vi "WILT Valve Test.vi"(0 "Water Valves Cluster":T8, 1 "Test Type":T7=enum."Full Valve Control", 2 "Operation Type":T11=enum."Operate As Stand-Alone EXE", 3 "Valve ON Time":dbl=100.0, 5 "Start Buttons Cluster":T9, 7 "Station Test State In":T5, 9 "Station Number":i32, 11 "Error In":errorcluster, 12 "Injection Times":T4, 13 "Day/Night Cycle":T10) -> (4 "Valve Actuation Complete":bool, 6 "Test Station Out":T5, 15 "Error Out":errorcluster)   [LabVIEW 2016] (continued)
                  tunnel: [T9 {"Start Button 21"=FALSE, "Start Button 22"=FALSE, "Start Button 23"=FALSE, "Start Button 24"=FALSE, "Start Button 25"=FALSE, "Start Button 26"=FALSE, "Start Button 27"=FALSE, "Start Button 28"=FALSE, "Start Button 29"=FALSE, "Start Button 30"=FALSE, "Start Button 31"=FALSE, "Start Button 32"=FALSE, "Start Button 33"=FALSE, "Start Button 34"=FALSE, "Start Button 35"=FALSE, "Start Button 36"=FALSE, "Start Button 37"=FALSE, "Start Button 38"=FALSE, "Start Button 39"=FALSE, "Start Button 40"=FALSE, "Start Button 41"=FALSE, "Start Button 42"=FALSE, "Start Button 43"=FALSE, "Start Button 44"=FALSE, "Start Button 12"=FALSE, "Start Button 11"=FALSE, "Start Button 10"=FALSE, "Start Button 9"=FALSE, "Start Button 8"=FALSE, "Start Button 7"=FALSE, "Start Button 6"=FALSE, "Start Button 5"=FALSE, "Start Button 4"=FALSE, "Start Button 3"=FALSE, "Start Button 2"=FALSE, "Start Button 1"=FALSE, "Start Button 20"=FALSE, "Start Button 19"=FALSE, "Start Button 18"=FALSE, "Start Button 17"=FALSE, "Start Button 16"=FALSE, "Start Button 15"=FALSE, "Start Button 14"=FALSE, "Start Button 13"=FALSE, "Start Button 45"=FALSE, "Start Button 46"=FALSE, "Start Button 47"=FALSE, "Start Button 48"=FALSE, "Start Button 49"=FALSE, "Start Button 50"=FALSE, "Start Button 51"=FALSE, "Start Button 52"=FALSE, "Start Button 53"=FALSE, "Start Button 54"=FALSE, "Start Button 55"=FALSE, "Start Button 56"=FALSE} ("Start Buttons Cluster") T9 {"Start Button 21"=FALSE, "Start Button 22"=FALSE, "Start Button 23"=FALSE, "Start Button 24"=FALSE, "Start Button 25"=FALSE, "Start Button 26"=FALSE, "Start Button 27"=FALSE, "Start Button 28"=FALSE, "Start Button 29"=FALSE, "Start Button 30"=FALSE, "Start Button 31"=FALSE, "Start Button 32"=FALSE, "Start Button 33"=FALSE, "Start Button 34"=FALSE, "Start Button 35"=FALSE, "Start Button 36"=FALSE, "Start Button 37"=FALSE, "Start Button 38"=FALSE, "Start Button 39"=FALSE, "Start Button 40"=FALSE, "Start Button 41"=FALSE, "Start Button 42"=FALSE, "Start Button 43"=FALSE, "Start Button 44"=FALSE, "Start Button 12"=FALSE, "Start Button 11"=FALSE, "Start Button 10"=FALSE, "Start Button 9"=FALSE, "Start Button 8"=FALSE, "Start Button 7"=FALSE, "Start Button 6"=FALSE, "Start Button 5"=FALSE, "Start Button 4"=FALSE, "Start Button 3"=FALSE, "Start Button 2"=FALSE, "Start Button 1"=FALSE, "Start Button 20"=FALSE, "Start Button 19"=FALSE, "Start Button 18"=FALSE, "Start Button 17"=FALSE, "Start Button 16"=FALSE, "Start Button 15"=FALSE, "Start Button 14"=FALSE, "Start Button 13"=FALSE, "Start Button 45"=FALSE, "Start Button 46"=FALSE, "Start Button 47"=FALSE, "Start Button 48"=FALSE, "Start Button 49"=FALSE, "Start Button 50"=FALSE, "Start Button 51"=FALSE, "Start Button 52"=FALSE, "Start Button 53"=FALSE, "Start Button 54"=FALSE, "Start Button 55"=FALSE, "Start Button 56"=FALSE} ("Start Buttons Cluster") w1471 w1474 w1478] -> w1458
                  frame "Water Injection 1 (On)", Default {
                    n436 = Bundle By Name(cluster=T8 {"Valve 1"=FALSE, "Valve 2"=FALSE, "Valve 3"=FALSE, "Valve 4"=FALSE, "Valve 5"=FALSE, "Valve 6"=FALSE, "Valve 7"=FALSE, "Valve 8"=FALSE, "Valve 9"=FALSE, "Valve 10"=FALSE, "Valve 11"=FALSE, "Valve 12"=FALSE, "Valve 13"=FALSE, "Valve 14"=FALSE, "Valve 15"=FALSE, "Valve 16"=FALSE, "Valve 17"=FALSE, "Valve 18"=FALSE, "Valve 19"=FALSE, "Valve 20"=FALSE, "Valve 21"=FALSE, "Valve 22"=FALSE, "Valve 23"=FALSE, "Valve 24"=FALSE, "Valve 25"=FALSE, "Valve 26"=FALSE, "Valve 27"=FALSE, "Valve 28"=FALSE, "Valve 29"=FALSE, "Valve 30"=FALSE, "Valve 31"=FALSE, "Valve 32"=FALSE, "Valve 33"=FALSE, "Valve 34"=FALSE, "Valve 35"=FALSE, "Valve 36"=FALSE, "Valve 37"=FALSE, "Valve 38"=FALSE, "Valve 39"=FALSE, "Valve 40"=FALSE, "Valve 41"=FALSE, "Valve 42"=FALSE, "Valve 43"=FALSE, "Valve 44"=FALSE, "Valve 45"=FALSE, "Valve 46"=FALSE, "Valve 47"=FALSE, "Valve 48"=FALSE, "Valve 49"=FALSE, "Valve 50"=FALSE, "Valve 51"=FALSE, "Valve 52"=FALSE, "Valve 53"=FALSE, "Valve 54"=FALSE, "Valve 55"=FALSE, "Valve 56"=FALSE} ("Water Valves Cluster"), "Valve 54"=TRUE ("Valve 1")) -> (w1463:T8)
                  }
                  frame "Drying Clothes 2" {
                    n437 = Bundle By Name(cluster=T8 {"Valve 1"=FALSE, "Valve 2"=FALSE, "Valve 3"=FALSE, "Valve 4"=FALSE, "Valve 5"=FALSE, "Valve 6"=FALSE, "Valve 7"=FALSE, "Valve 8"=FALSE, "Valve 9"=FALSE, "Valve 10"=FALSE, "Valve 11"=FALSE, "Valve 12"=FALSE, "Valve 13"=FALSE, "Valve 14"=FALSE, "Valve 15"=FALSE, "Valve 16"=FALSE, "Valve 17"=FALSE, "Valve 18"=FALSE, "Valve 19"=FALSE, "Valve 20"=FALSE, "Valve 21"=FALSE, "Valve 22"=FALSE, "Valve 23"=FALSE, "Valve 24"=FALSE, "Valve 25"=FALSE, "Valve 26"=FALSE, "Valve 27"=FALSE, "Valve 28"=FALSE, "Valve 29"=FALSE, "Valve 30"=FALSE, "Valve 31"=FALSE, "Valve 32"=FALSE, "Valve 33"=FALSE, "Valve 34"=FALSE, "Valve 35"=FALSE, "Valve 36"=FALSE, "Valve 37"=FALSE, "Valve 38"=FALSE, "Valve 39"=FALSE, "Valve 40"=FALSE, "Valve 41"=FALSE, "Valve 42"=FALSE, "Valve 43"=FALSE, "Valve 44"=FALSE, "Valve 45"=FALSE, "Valve 46"=FALSE, "Valve 47"=FALSE, "Valve 48"=FALSE, "Valve 49"=FALSE, "Valve 50"=FALSE, "Valve 51"=FALSE, "Valve 52"=FALSE, "Valve 53"=FALSE, "Valve 54"=FALSE, "Valve 55"=FALSE, "Valve 56"=FALSE} ("Water Valves Cluster"), "Valve 54"=TRUE ("Valve 1")) -> (w1467:T8)
                  }
                  frame "Sending Start Stop CMD" {
                    n438 = Bundle By Name(cluster=T9 {"Start Button 21"=FALSE, "Start Button 22"=FALSE, "Start Button 23"=FALSE, "Start Button 24"=FALSE, "Start Button 25"=FALSE, "Start Button 26"=FALSE, "Start Button 27"=FALSE, "Start Button 28"=FALSE, "Start Button 29"=FALSE, "Start Button 30"=FALSE, "Start Button 31"=FALSE, "Start Button 32"=FALSE, "Start Button 33"=FALSE, "Start Button 34"=FALSE, "Start Button 35"=FALSE, "Start Button 36"=FALSE, "Start Button 37"=FALSE, "Start Button 38"=FALSE, "Start Button 39"=FALSE, "Start Button 40"=FALSE, "Start Button 41"=FALSE, "Start Button 42"=FALSE, "Start Button 43"=FALSE, "Start Button 44"=FALSE, "Start Button 12"=FALSE, "Start Button 11"=FALSE, "Start Button 10"=FALSE, "Start Button 9"=FALSE, "Start Button 8"=FALSE, "Start Button 7"=FALSE, "Start Button 6"=FALSE, "Start Button 5"=FALSE, "Start Button 4"=FALSE, "Start Button 3"=FALSE, "Start Button 2"=FALSE, "Start Button 1"=FALSE, "Start Button 20"=FALSE, "Start Button 19"=FALSE, "Start Button 18"=FALSE, "Start Button 17"=FALSE, "Start Button 16"=FALSE, "Start Button 15"=FALSE, "Start Button 14"=FALSE, "Start Button 13"=FALSE, "Start Button 45"=FALSE, "Start Button 46"=FALSE, "Start Button 47"=FALSE, "Start Button 48"=FALSE, "Start Button 49"=FALSE, "Start Button 50"=FALSE, "Start Button 51"=FALSE, "Start Button 52"=FALSE, "Start Button 53"=FALSE, "Start Button 54"=FALSE, "Start Button 55"=FALSE, "Start Button 56"=FALSE} ("Start Buttons Cluster"), "Start Button 54"=TRUE ("Start Button 21")) -> (w1471:T9)
                  }
                  frame "Sending Start Stop CMD 2" {
                    n439 = Bundle By Name(cluster=T9 {"Start Button 21"=FALSE, "Start Button 22"=FALSE, "Start Button 23"=FALSE, "Start Button 24"=FALSE, "Start Button 25"=FALSE, "Start Button 26"=FALSE, "Start Button 27"=FALSE, "Start Button 28"=FALSE, "Start Button 29"=FALSE, "Start Button 30"=FALSE, "Start Button 31"=FALSE, "Start Button 32"=FALSE, "Start Button 33"=FALSE, "Start Button 34"=FALSE, "Start Button 35"=FALSE, "Start Button 36"=FALSE, "Start Button 37"=FALSE, "Start Button 38"=FALSE, "Start Button 39"=FALSE, "Start Button 40"=FALSE, "Start Button 41"=FALSE, "Start Button 42"=FALSE, "Start Button 43"=FALSE, "Start Button 44"=FALSE, "Start Button 12"=FALSE, "Start Button 11"=FALSE, "Start Button 10"=FALSE, "Start Button 9"=FALSE, "Start Button 8"=FALSE, "Start Button 7"=FALSE, "Start Button 6"=FALSE, "Start Button 5"=FALSE, "Start Button 4"=FALSE, "Start Button 3"=FALSE, "Start Button 2"=FALSE, "Start Button 1"=FALSE, "Start Button 20"=FALSE, "Start Button 19"=FALSE, "Start Button 18"=FALSE, "Start Button 17"=FALSE, "Start Button 16"=FALSE, "Start Button 15"=FALSE, "Start Button 14"=FALSE, "Start Button 13"=FALSE, "Start Button 45"=FALSE, "Start Button 46"=FALSE, "Start Button 47"=FALSE, "Start Button 48"=FALSE, "Start Button 49"=FALSE, "Start Button 50"=FALSE, "Start Button 51"=FALSE, "Start Button 52"=FALSE, "Start Button 53"=FALSE, "Start Button 54"=FALSE, "Start Button 55"=FALSE, "Start Button 56"=FALSE} ("Start Buttons Cluster"), "Start Button 54"=TRUE ("Start Button 21")) -> (w1474:T9)
                  }
                  frame "Sending Start Stop CMD 3" {
                    n440 = Bundle By Name(cluster=T9 {"Start Button 21"=FALSE, "Start Button 22"=FALSE, "Start Button 23"=FALSE, "Start Button 24"=FALSE, "Start Button 25"=FALSE, "Start Button 26"=FALSE, "Start Button 27"=FALSE, "Start Button 28"=FALSE, "Start Button 29"=FALSE, "Start Button 30"=FALSE, "Start Button 31"=FALSE, "Start Button 32"=FALSE, "Start Button 33"=FALSE, "Start Button 34"=FALSE, "Start Button 35"=FALSE, "Start Button 36"=FALSE, "Start Button 37"=FALSE, "Start Button 38"=FALSE, "Start Button 39"=FALSE, "Start Button 40"=FALSE, "Start Button 41"=FALSE, "Start Button 42"=FALSE, "Start Button 43"=FALSE, "Start Button 44"=FALSE, "Start Button 12"=FALSE, "Start Button 11"=FALSE, "Start Button 10"=FALSE, "Start Button 9"=FALSE, "Start Button 8"=FALSE, "Start Button 7"=FALSE, "Start Button 6"=FALSE, "Start Button 5"=FALSE, "Start Button 4"=FALSE, "Start Button 3"=FALSE, "Start Button 2"=FALSE, "Start Button 1"=FALSE, "Start Button 20"=FALSE, "Start Button 19"=FALSE, "Start Button 18"=FALSE, "Start Button 17"=FALSE, "Start Button 16"=FALSE, "Start Button 15"=FALSE, "Start Button 14"=FALSE, "Start Button 13"=FALSE, "Start Button 45"=FALSE, "Start Button 46"=FALSE, "Start Button 47"=FALSE, "Start Button 48"=FALSE, "Start Button 49"=FALSE, "Start Button 50"=FALSE, "Start Button 51"=FALSE, "Start Button 52"=FALSE, "Start Button 53"=FALSE, "Start Button 54"=FALSE, "Start Button 55"=FALSE, "Start Button 56"=FALSE} ("Start Buttons Cluster"), "Start Button 54"=TRUE ("Start Button 21")) -> (w1478:T9)
                  }
                }
              }
              frame 55 {
                n441 = Unbundle By Name(w1485) -> ("Station Test State 55"=w1484:T6)
                n442 = case shown="\"Sending Start Stop CMD 3\"" w1484 {
                  tunnel: [w1487 w1491 T8 {"Valve 1"=FALSE, "Valve 2"=FALSE, "Valve 3"=FALSE, "Valve 4"=FALSE, "Valve 5"=FALSE, "Valve 6"=FALSE, "Valve 7"=FALSE, "Valve 8"=FALSE, "Valve 9"=FALSE, "Valve 10"=FALSE, "Valve 11"=FALSE, "Valve 12"=FALSE, "Valve 13"=FALSE, "Valve 14"=FALSE, "Valve 15"=FALSE, "Valve 16"=FALSE, "Valve 17"=FALSE, "Valve 18"=FALSE, "Valve 19"=FALSE, "Valve 20"=FALSE, "Valve 21"=FALSE, "Valve 22"=FALSE, "Valve 23"=FALSE, "Valve 24"=FALSE, "Valve 25"=FALSE, "Valve 26"=FALSE, "Valve 27"=FALSE, "Valve 28"=FALSE, "Valve 29"=FALSE, "Valve 30"=FALSE, "Valve 31"=FALSE, "Valve 32"=FALSE, "Valve 33"=FALSE, "Valve 34"=FALSE, "Valve 35"=FALSE, "Valve 36"=FALSE, "Valve 37"=FALSE, "Valve 38"=FALSE, "Valve 39"=FALSE, "Valve 40"=FALSE, "Valve 41"=FALSE, "Valve 42"=FALSE, "Valve 43"=FALSE, "Valve 44"=FALSE, "Valve 45"=FALSE, "Valve 46"=FALSE, "Valve 47"=FALSE, "Valve 48"=FALSE, "Valve 49"=FALSE, "Valve 50"=FALSE, "Valve 51"=FALSE, "Valve 52"=FALSE, "Valve 53"=FALSE, "Valve 54"=FALSE, "Valve 55"=FALSE, "Valve 56"=FALSE} ("Water Valves Cluster") T8 {"Valve 1"=FALSE, "Valve 2"=FALSE, "Valve 3"=FALSE, "Valve 4"=FALSE, "Valve 5"=FALSE, "Valve 6"=FALSE, "Valve 7"=FALSE, "Valve 8"=FALSE, "Valve 9"=FALSE, "Valve 10"=FALSE, "Valve 11"=FALSE, "Valve 12"=FALSE, "Valve 13"=FALSE, "Valve 14"=FALSE, "Valve 15"=FALSE, "Valve 16"=FALSE, "Valve 17"=FALSE, "Valve 18"=FALSE, "Valve 19"=FALSE, "Valve 20"=FALSE, "Valve 21"=FALSE, "Valve 22"=FALSE, "Valve 23"=FALSE, "Valve 24"=FALSE, "Valve 25"=FALSE, "Valve 26"=FALSE, "Valve 27"=FALSE, "Valve 28"=FALSE, "Valve 29"=FALSE, "Valve 30"=FALSE, "Valve 31"=FALSE, "Valve 32"=FALSE, "Valve 33"=FALSE, "Valve 34"=FALSE, "Valve 35"=FALSE, "Valve 36"=FALSE, "Valve 37"=FALSE, "Valve 38"=FALSE, "Valve 39"=FALSE, "Valve 40"=FALSE, "Valve 41"=FALSE, "Valve 42"=FALSE, "Valve 43"=FALSE, "Valve 44"=FALSE, "Valve 45"=FALSE, "Valve 46"=FALSE, "Valve 47"=FALSE, "Valve 48"=FALSE, "Valve 49"=FALSE, "Valve 50"=FALSE, "Valve 51"=FALSE, "Valve 52"=FALSE, "Valve 53"=FALSE, "Valve 54"=FALSE, "Valve 55"=FALSE, "Valve 56"=FALSE} ("Water Valves Cluster") T8 {"Valve 1"=FALSE, "Valve 2"=FALSE, "Valve 3"=FALSE, "Valve 4"=FALSE, "Valve 5"=FALSE, "Valve 6"=FALSE, "Valve 7"=FALSE, "Valve 8"=FALSE, "Valve 9"=FALSE, "Valve 10"=FALSE, "Valve 11"=FALSE, "Valve 12"=FALSE, "Valve 13"=FALSE, "Valve 14"=FALSE, "Valve 15"=FALSE, "Valve 16"=FALSE, "Valve 17"=FALSE, "Valve 18"=FALSE, "Valve 19"=FALSE, "Valve 20"=FALSE, "Valve 21"=FALSE, "Valve 22"=FALSE, "Valve 23"=FALSE, "Valve 24"=FALSE, "Valve 25"=FALSE, "Valve 26"=FALSE, "Valve 27"=FALSE, "Valve 28"=FALSE, "Valve 29"=FALSE, "Valve 30"=FALSE, "Valve 31"=FALSE, "Valve 32"=FALSE, "Valve 33"=FALSE, "Valve 34"=FALSE, "Valve 35"=FALSE, "Valve 36"=FALSE, "Valve 37"=FALSE, "Valve 38"=FALSE, "Valve 39"=FALSE, "Valve 40"=FALSE, "Valve 41"=FALSE, "Valve 42"=FALSE, "Valve 43"=FALSE, "Valve 44"=FALSE, "Valve 45"=FALSE, "Valve 46"=FALSE, "Valve 47"=FALSE, "Valve 48"=FALSE, "Valve 49"=FALSE, "Valve 50"=FALSE, "Valve 51"=FALSE, "Valve 52"=FALSE, "Valve 53"=FALSE, "Valve 54"=FALSE, "Valve 55"=FALSE, "Valve 56"=FALSE} ("Water Valves Cluster")] -> w1483
                  tunnel: [T9 {"Start Button 21"=FALSE, "Start Button 22"=FALSE, "Start Button 23"=FALSE, "Start Button 24"=FALSE, "Start Button 25"=FALSE, "Start Button 26"=FALSE, "Start Button 27"=FALSE, "Start Button 28"=FALSE, "Start Button 29"=FALSE, "Start Button 30"=FALSE, "Start Button 31"=FALSE, "Start Button 32"=FALSE, "Start Button 33"=FALSE, "Start Button 34"=FALSE, "Start Button 35"=FALSE, "Start Button 36"=FALSE, "Start Button 37"=FALSE, "Start Button 38"=FALSE, "Start Button 39"=FALSE, "Start Button 40"=FALSE, "Start Button 41"=FALSE, "Start Button 42"=FALSE, "Start Button 43"=FALSE, "Start Button 44"=FALSE, "Start Button 12"=FALSE, "Start Button 11"=FALSE, "Start Button 10"=FALSE, "Start Button 9"=FALSE, "Start Button 8"=FALSE, "Start Button 7"=FALSE, "Start Button 6"=FALSE, "Start Button 5"=FALSE, "Start Button 4"=FALSE, "Start Button 3"=FALSE, "Start Button 2"=FALSE, "Start Button 1"=FALSE, "Start Button 20"=FALSE, "Start Button 19"=FALSE, "Start Button 18"=FALSE, "Start Button 17"=FALSE, "Start Button 16"=FALSE, "Start Button 15"=FALSE, "Start Button 14"=FALSE, "Start Button 13"=FALSE, "Start Button 45"=FALSE, "Start Button 46"=FALSE, "Start Button 47"=FALSE, "Start Button 48"=FALSE, "Start Button 49"=FALSE, "Start Button 50"=FALSE, "Start Button 51"=FALSE, "Start Button 52"=FALSE, "Start Button 53"=FALSE, "Start Button 54"=FALSE, "Start Button 55"=FALSE, "Start Button 56"=FALSE} ("Start Buttons Cluster") T9 {"Start Button 21"=FALSE, "Start Button 22"=FALSE, "Start Button 23"=FALSE, "Start Button 24"=FALSE, "Start Button 25"=FALSE, "Start Button 26"=FALSE, "Start Button 27"=FALSE, "Start Button 28"=FALSE, "Start Button 29"=FALSE, "Start Button 30"=FALSE, "Start Button 31"=FALSE, "Start Button 32"=FALSE, "Start Button 33"=FALSE, "Start Button 34"=FALSE, "Start Button 35"=FALSE, "Start Button 36"=FALSE, "Start Button 37"=FALSE, "Start Button 38"=FALSE, "Start Button 39"=FALSE, "Start Button 40"=FALSE, "Start Button 41"=FALSE, "Start Button 42"=FALSE, "Start Button 43"=FALSE, "Start Button 44"=FALSE, "Start Button 12"=FALSE, "Start Button 11"=FALSE, "Start Button 10"=FALSE, "Start Button 9"=FALSE, "Start Button 8"=FALSE, "Start Button 7"=FALSE, "Start Button 6"=FALSE, "Start Button 5"=FALSE, "Start Button 4"=FALSE, "Start Button 3"=FALSE, "Start Button 2"=FALSE, "Start Button 1"=FALSE, "Start Button 20"=FALSE, "Start Button 19"=FALSE, "Start Button 18"=FALSE, "Start Button 17"=FALSE, "Start Button 16"=FALSE, "Start Button 15"=FALSE, "Start Button 14"=FALSE, "Start Button 13"=FALSE, "Start Button 45"=FALSE, "Start Button 46"=FALSE, "Start Button 47"=FALSE, "Start Button 48"=FALSE, "Start Button 49"=FALSE, "Start Button 50"=FALSE, "Start Button 51"=FALSE, "Start Button 52"=FALSE, "Start Button 53"=FALSE, "Start Button 54"=FALSE, "Start Button 55"=FALSE, "Start Button 56"=FALSE} ("Start Buttons Cluster") w1495 w1498 w1502] -> w1482
                  frame "Water Injection 1 (On)", Default {
                    n443 = Bundle By Name(cluster=T8 {"Valve 1"=FALSE, "Valve 2"=FALSE, "Valve 3"=FALSE, "Valve 4"=FALSE, "Valve 5"=FALSE, "Valve 6"=FALSE, "Valve 7"=FALSE, "Valve 8"=FALSE, "Valve 9"=FALSE, "Valve 10"=FALSE, "Valve 11"=FALSE, "Valve 12"=FALSE, "Valve 13"=FALSE, "Valve 14"=FALSE, "Valve 15"=FALSE, "Valve 16"=FALSE, "Valve 17"=FALSE, "Valve 18"=FALSE, "Valve 19"=FALSE, "Valve 20"=FALSE, "Valve 21"=FALSE, "Valve 22"=FALSE, "Valve 23"=FALSE, "Valve 24"=FALSE, "Valve 25"=FALSE, "Valve 26"=FALSE, "Valve 27"=FALSE, "Valve 28"=FALSE, "Valve 29"=FALSE, "Valve 30"=FALSE, "Valve 31"=FALSE, "Valve 32"=FALSE, "Valve 33"=FALSE, "Valve 34"=FALSE, "Valve 35"=FALSE, "Valve 36"=FALSE, "Valve 37"=FALSE, "Valve 38"=FALSE, "Valve 39"=FALSE, "Valve 40"=FALSE, "Valve 41"=FALSE, "Valve 42"=FALSE, "Valve 43"=FALSE, "Valve 44"=FALSE, "Valve 45"=FALSE, "Valve 46"=FALSE, "Valve 47"=FALSE, "Valve 48"=FALSE, "Valve 49"=FALSE, "Valve 50"=FALSE, "Valve 51"=FALSE, "Valve 52"=FALSE, "Valve 53"=FALSE, "Valve 54"=FALSE, "Valve 55"=FALSE, "Valve 56"=FALSE} ("Water Valves Cluster"), "Valve 55"=TRUE ("Valve 1")) -> (w1487:T8)
                  }
                  frame "Drying Clothes 2" {
                    n444 = Bundle By Name(cluster=T8 {"Valve 1"=FALSE, "Valve 2"=FALSE, "Valve 3"=FALSE, "Valve 4"=FALSE, "Valve 5"=FALSE, "Valve 6"=FALSE, "Valve 7"=FALSE, "Valve 8"=FALSE, "Valve 9"=FALSE, "Valve 10"=FALSE, "Valve 11"=FALSE, "Valve 12"=FALSE, "Valve 13"=FALSE, "Valve 14"=FALSE, "Valve 15"=FALSE, "Valve 16"=FALSE, "Valve 17"=FALSE, "Valve 18"=FALSE, "Valve 19"=FALSE, "Valve 20"=FALSE, "Valve 21"=FALSE, "Valve 22"=FALSE, "Valve 23"=FALSE, "Valve 24"=FALSE, "Valve 25"=FALSE, "Valve 26"=FALSE, "Valve 27"=FALSE, "Valve 28"=FALSE, "Valve 29"=FALSE, "Valve 30"=FALSE, "Valve 31"=FALSE, "Valve 32"=FALSE, "Valve 33"=FALSE, "Valve 34"=FALSE, "Valve 35"=FALSE, "Valve 36"=FALSE, "Valve 37"=FALSE, "Valve 38"=FALSE, "Valve 39"=FALSE, "Valve 40"=FALSE, "Valve 41"=FALSE, "Valve 42"=FALSE, "Valve 43"=FALSE, "Valve 44"=FALSE, "Valve 45"=FALSE, "Valve 46"=FALSE, "Valve 47"=FALSE, "Valve 48"=FALSE, "Valve 49"=FALSE, "Valve 50"=FALSE, "Valve 51"=FALSE, "Valve 52"=FALSE, "Valve 53"=FALSE, "Valve 54"=FALSE, "Valve 55"=FALSE, "Valve 56"=FALSE} ("Water Valves Cluster"), "Valve 55"=TRUE ("Valve 1")) -> (w1491:T8)
                  }
                  frame "Sending Start Stop CMD" {
                    n445 = Bundle By Name(cluster=T9 {"Start Button 21"=FALSE, "Start Button 22"=FALSE, "Start Button 23"=FALSE, "Start Button 24"=FALSE, "Start Button 25"=FALSE, "Start Button 26"=FALSE, "Start Button 27"=FALSE, "Start Button 28"=FALSE, "Start Button 29"=FALSE, "Start Button 30"=FALSE, "Start Button 31"=FALSE, "Start Button 32"=FALSE, "Start Button 33"=FALSE, "Start Button 34"=FALSE, "Start Button 35"=FALSE, "Start Button 36"=FALSE, "Start Button 37"=FALSE, "Start Button 38"=FALSE, "Start Button 39"=FALSE, "Start Button 40"=FALSE, "Start Button 41"=FALSE, "Start Button 42"=FALSE, "Start Button 43"=FALSE, "Start Button 44"=FALSE, "Start Button 12"=FALSE, "Start Button 11"=FALSE, "Start Button 10"=FALSE, "Start Button 9"=FALSE, "Start Button 8"=FALSE, "Start Button 7"=FALSE, "Start Button 6"=FALSE, "Start Button 5"=FALSE, "Start Button 4"=FALSE, "Start Button 3"=FALSE, "Start Button 2"=FALSE, "Start Button 1"=FALSE, "Start Button 20"=FALSE, "Start Button 19"=FALSE, "Start Button 18"=FALSE, "Start Button 17"=FALSE, "Start Button 16"=FALSE, "Start Button 15"=FALSE, "Start Button 14"=FALSE, "Start Button 13"=FALSE, "Start Button 45"=FALSE, "Start Button 46"=FALSE, "Start Button 47"=FALSE, "Start Button 48"=FALSE, "Start Button 49"=FALSE, "Start Button 50"=FALSE, "Start Button 51"=FALSE, "Start Button 52"=FALSE, "Start Button 53"=FALSE, "Start Button 54"=FALSE, "Start Button 55"=FALSE, "Start Button 56"=FALSE} ("Start Buttons Cluster"), "Start Button 55"=TRUE ("Start Button 21")) -> (w1495:T9)
                  }
                  frame "Sending Start Stop CMD 2" {
                    n446 = Bundle By Name(cluster=T9 {"Start Button 21"=FALSE, "Start Button 22"=FALSE, "Start Button 23"=FALSE, "Start Button 24"=FALSE, "Start Button 25"=FALSE, "Start Button 26"=FALSE, "Start Button 27"=FALSE, "Start Button 28"=FALSE, "Start Button 29"=FALSE, "Start Button 30"=FALSE, "Start Button 31"=FALSE, "Start Button 32"=FALSE, "Start Button 33"=FALSE, "Start Button 34"=FALSE, "Start Button 35"=FALSE, "Start Button 36"=FALSE, "Start Button 37"=FALSE, "Start Button 38"=FALSE, "Start Button 39"=FALSE, "Start Button 40"=FALSE, "Start Button 41"=FALSE, "Start Button 42"=FALSE, "Start Button 43"=FALSE, "Start Button 44"=FALSE, "Start Button 12"=FALSE, "Start Button 11"=FALSE, "Start Button 10"=FALSE, "Start Button 9"=FALSE, "Start Button 8"=FALSE, "Start Button 7"=FALSE, "Start Button 6"=FALSE, "Start Button 5"=FALSE, "Start Button 4"=FALSE, "Start Button 3"=FALSE, "Start Button 2"=FALSE, "Start Button 1"=FALSE, "Start Button 20"=FALSE, "Start Button 19"=FALSE, "Start Button 18"=FALSE, "Start Button 17"=FALSE, "Start Button 16"=FALSE, "Start Button 15"=FALSE, "Start Button 14"=FALSE, "Start Button 13"=FALSE, "Start Button 45"=FALSE, "Start Button 46"=FALSE, "Start Button 47"=FALSE, "Start Button 48"=FALSE, "Start Button 49"=FALSE, "Start Button 50"=FALSE, "Start Button 51"=FALSE, "Start Button 52"=FALSE, "Start Button 53"=FALSE, "Start Button 54"=FALSE, "Start Button 55"=FALSE, "Start Button 56"=FALSE} ("Start Buttons Cluster"), "Start Button 55"=TRUE ("Start Button 21")) -> (w1498:T9)
                  }
                  frame "Sending Start Stop CMD 3" {
                    n447 = Bundle By Name(cluster=T9 {"Start Button 21"=FALSE, "Start Button 22"=FALSE, "Start Button 23"=FALSE, "Start Button 24"=FALSE, "Start Button 25"=FALSE, "Start Button 26"=FALSE, "Start Button 27"=FALSE, "Start Button 28"=FALSE, "Start Button 29"=FALSE, "Start Button 30"=FALSE, "Start Button 31"=FALSE, "Start Button 32"=FALSE, "Start Button 33"=FALSE, "Start Button 34"=FALSE, "Start Button 35"=FALSE, "Start Button 36"=FALSE, "Start Button 37"=FALSE, "Start Button 38"=FALSE, "Start Button 39"=FALSE, "Start Button 40"=FALSE, "Start Button 41"=FALSE, "Start Button 42"=FALSE, "Start Button 43"=FALSE, "Start Button 44"=FALSE, "Start Button 12"=FALSE, "Start Button 11"=FALSE, "Start Button 10"=FALSE, "Start Button 9"=FALSE, "Start Button 8"=FALSE, "Start Button 7"=FALSE, "Start Button 6"=FALSE, "Start Button 5"=FALSE, "Start Button 4"=FALSE, "Start Button 3"=FALSE, "Start Button 2"=FALSE, "Start Button 1"=FALSE, "Start Button 20"=FALSE, "Start Button 19"=FALSE, "Start Button 18"=FALSE, "Start Button 17"=FALSE, "Start Button 16"=FALSE, "Start Button 15"=FALSE, "Start Button 14"=FALSE, "Start Button 13"=FALSE, "Start Button 45"=FALSE, "Start Button 46"=FALSE, "Start Button 47"=FALSE, "Start Button 48"=FALSE, "Start Button 49"=FALSE, "Start Button 50"=FALSE, "Start Button 51"=FALSE, "Start Button 52"=FALSE, "Start Button 53"=FALSE, "Start Button 54"=FALSE, "Start Button 55"=FALSE, "Start Button 56"=FALSE} ("Start Buttons Cluster"), "Start Button 55"=TRUE ("Start Button 21")) -> (w1502:T9)
                  }
                }
              }
              frame 56 {
                n448 = Unbundle By Name(w1509) -> ("Station Test State 56"=w1508:T6)
                n449 = case shown="\"Water Injection 1 (On)\", Default" w1508 {
                  tunnel: [w1511 w1515 T8 {"Valve 1"=FALSE, "Valve 2"=FALSE, "Valve 3"=FALSE, "Valve 4"=FALSE, "Valve 5"=FALSE, "Valve 6"=FALSE, "Valve 7"=FALSE, "Valve 8"=FALSE, "Valve 9"=FALSE, "Valve 10"=FALSE, "Valve 11"=FALSE, "Valve 12"=FALSE, "Valve 13"=FALSE, "Valve 14"=FALSE, "Valve 15"=FALSE, "Valve 16"=FALSE, "Valve 17"=FALSE, "Valve 18"=FALSE, "Valve 19"=FALSE, "Valve 20"=FALSE, "Valve 21"=FALSE, "Valve 22"=FALSE, "Valve 23"=FALSE, "Valve 24"=FALSE, "Valve 25"=FALSE, "Valve 26"=FALSE, "Valve 27"=FALSE, "Valve 28"=FALSE, "Valve 29"=FALSE, "Valve 30"=FALSE, "Valve 31"=FALSE, "Valve 32"=FALSE, "Valve 33"=FALSE, "Valve 34"=FALSE, "Valve 35"=FALSE, "Valve 36"=FALSE, "Valve 37"=FALSE, "Valve 38"=FALSE, "Valve 39"=FALSE, "Valve 40"=FALSE, "Valve 41"=FALSE, "Valve 42"=FALSE, "Valve 43"=FALSE, "Valve 44"=FALSE, "Valve 45"=FALSE, "Valve 46"=FALSE, "Valve 47"=FALSE, "Valve 48"=FALSE, "Valve 49"=FALSE, "Valve 50"=FALSE, "Valve 51"=FALSE, "Valve 52"=FALSE, "Valve 53"=FALSE, "Valve 54"=FALSE, "Valve 55"=FALSE, "Valve 56"=FALSE} ("Water Valves Cluster") T8 {"Valve 1"=FALSE, "Valve 2"=FALSE, "Valve 3"=FALSE, "Valve 4"=FALSE, "Valve 5"=FALSE, "Valve 6"=FALSE, "Valve 7"=FALSE, "Valve 8"=FALSE, "Valve 9"=FALSE, "Valve 10"=FALSE, "Valve 11"=FALSE, "Valve 12"=FALSE, "Valve 13"=FALSE, "Valve 14"=FALSE, "Valve 15"=FALSE, "Valve 16"=FALSE, "Valve 17"=FALSE, "Valve 18"=FALSE, "Valve 19"=FALSE, "Valve 20"=FALSE, "Valve 21"=FALSE, "Valve 22"=FALSE, "Valve 23"=FALSE, "Valve 24"=FALSE, "Valve 25"=FALSE, "Valve 26"=FALSE, "Valve 27"=FALSE, "Valve 28"=FALSE, "Valve 29"=FALSE, "Valve 30"=FALSE, "Valve 31"=FALSE, "Valve 32"=FALSE, "Valve 33"=FALSE, "Valve 34"=FALSE, "Valve 35"=FALSE, "Valve 36"=FALSE, "Valve 37"=FALSE, "Valve 38"=FALSE, "Valve 39"=FALSE, "Valve 40"=FALSE, "Valve 41"=FALSE, "Valve 42"=FALSE, "Valve 43"=FALSE, "Valve 44"=FALSE, "Valve 45"=FALSE, "Valve 46"=FALSE, "Valve 47"=FALSE, "Valve 48"=FALSE, "Valve 49"=FALSE, "Valve 50"=FALSE, "Valve 51"=FALSE, "Valve 52"=FALSE, "Valve 53"=FALSE, "Valve 54"=FALSE, "Valve 55"=FALSE, "Valve 56"=FALSE} ("Water Valves Cluster") T8 {"Valve 1"=FALSE, "Valve 2"=FALSE, "Valve 3"=FALSE, "Valve 4"=FALSE, "Valve 5"=FALSE, "Valve 6"=FALSE, "Valve 7"=FALSE, "Valve 8"=FALSE, "Valve 9"=FALSE, "Valve 10"=FALSE, "Valve 11"=FALSE, "Valve 12"=FALSE, "Valve 13"=FALSE, "Valve 14"=FALSE, "Valve 15"=FALSE, "Valve 16"=FALSE, "Valve 17"=FALSE, "Valve 18"=FALSE, "Valve 19"=FALSE, "Valve 20"=FALSE, "Valve 21"=FALSE, "Valve 22"=FALSE, "Valve 23"=FALSE, "Valve 24"=FALSE, "Valve 25"=FALSE, "Valve 26"=FALSE, "Valve 27"=FALSE, "Valve 28"=FALSE, "Valve 29"=FALSE, "Valve 30"=FALSE, "Valve 31"=FALSE, "Valve 32"=FALSE, "Valve 33"=FALSE, "Valve 34"=FALSE, "Valve 35"=FALSE, "Valve 36"=FALSE, "Valve 37"=FALSE, "Valve 38"=FALSE, "Valve 39"=FALSE, "Valve 40"=FALSE, "Valve 41"=FALSE, "Valve 42"=FALSE, "Valve 43"=FALSE, "Valve 44"=FALSE, "Valve 45"=FALSE, "Valve 46"=FALSE, "Valve 47"=FALSE, "Valve 48"=FALSE, "Valve 49"=FALSE, "Valve 50"=FALSE, "Valve 51"=FALSE, "Valve 52"=FALSE, "Valve 53"=FALSE, "Valve 54"=FALSE, "Valve 55"=FALSE, "Valve 56"=FALSE} ("Water Valves Cluster")] -> w1507
                  tunnel: [T9 {"Start Button 21"=FALSE, "Start Button 22"=FALSE, "Start Button 23"=FALSE, "Start Button 24"=FALSE, "Start Button 25"=FALSE, "Start Button 26"=FALSE, "Start Button 27"=FALSE, "Start Button 28"=FALSE, "Start Button 29"=FALSE, "Start Button 30"=FALSE, "Start Button 31"=FALSE, "Start Button 32"=FALSE, "Start Button 33"=FALSE, "Start Button 34"=FALSE, "Start Button 35"=FALSE, "Start Button 36"=FALSE, "Start Button 37"=FALSE, "Start Button 38"=FALSE, "Start Button 39"=FALSE, "Start Button 40"=FALSE, "Start Button 41"=FALSE, "Start Button 42"=FALSE, "Start Button 43"=FALSE, "Start Button 44"=FALSE, "Start Button 12"=FALSE, "Start Button 11"=FALSE, "Start Button 10"=FALSE, "Start Button 9"=FALSE, "Start Button 8"=FALSE, "Start Button 7"=FALSE, "Start Button 6"=FALSE, "Start Button 5"=FALSE, "Start Button 4"=FALSE, "Start Button 3"=FALSE, "Start Button 2"=FALSE, "Start Button 1"=FALSE, "Start Button 20"=FALSE, "Start Button 19"=FALSE, "Start Button 18"=FALSE, "Start Button 17"=FALSE, "Start Button 16"=FALSE, "Start Button 15"=FALSE, "Start Button 14"=FALSE, "Start Button 13"=FALSE, "Start Button 45"=FALSE, "Start Button 46"=FALSE, "Start Button 47"=FALSE, "Start Button 48"=FALSE, "Start Button 49"=FALSE, "Start Button 50"=FALSE, "Start Button 51"=FALSE, "Start Button 52"=FALSE, "Start Button 53"=FALSE, "Start Button 54"=FALSE, "Start Button 55"=FALSE, "Start Button 56"=FALSE} ("Start Buttons Cluster") T9 {"Start Button 21"=FALSE, "Start Button 22"=FALSE, "Start Button 23"=FALSE, "Start Button 24"=FALSE, "Start Button 25"=FALSE, "Start Button 26"=FALSE, "Start Button 27"=FALSE, "Start Button 28"=FALSE, "Start Button 29"=FALSE, "Start Button 30"=FALSE, "Start Button 31"=FALSE, "Start Button 32"=FALSE, "Start Button 33"=FALSE, "Start Button 34"=FALSE, "Start Button 35"=FALSE, "Start Button 36"=FALSE, "Start Button 37"=FALSE, "Start Button 38"=FALSE, "Start Button 39"=FALSE, "Start Button 40"=FALSE, "Start Button 41"=FALSE, "Start Button 42"=FALSE, "Start Button 43"=FALSE, "Start Button 44"=FALSE, "Start Button 12"=FALSE, "Start Button 11"=FALSE, "Start Button 10"=FALSE, "Start Button 9"=FALSE, "Start Button 8"=FALSE, "Start Button 7"=FALSE, "Start Button 6"=FALSE, "Start Button 5"=FALSE, "Start Button 4"=FALSE, "Start Button 3"=FALSE, "Start Button 2"=FALSE, "Start Button 1"=FALSE, "Start Button 20"=FALSE, "Start Button 19"=FALSE, "Start Button 18"=FALSE, "Start Button 17"=FALSE, "Start Button 16"=FALSE, "Start Button 15"=FALSE, "Start Button 14"=FALSE, "Start Button 13"=FALSE, "Start Button 45"=FALSE, "Start Button 46"=FALSE, "Start Button 47"=FALSE, "Start Button 48"=FALSE, "Start Button 49"=FALSE, "Start Button 50"=FALSE, "Start Button 51"=FALSE, "Start Button 52"=FALSE, "Start Button 53"=FALSE, "Start Button 54"=FALSE, "Start Button 55"=FALSE, "Start Button 56"=FALSE} ("Start Buttons Cluster") w1519 w1522 w1526] -> w1506
                  frame "Water Injection 1 (On)", Default {
                    n450 = Bundle By Name(cluster=T8 {"Valve 1"=FALSE, "Valve 2"=FALSE, "Valve 3"=FALSE, "Valve 4"=FALSE, "Valve 5"=FALSE, "Valve 6"=FALSE, "Valve 7"=FALSE, "Valve 8"=FALSE, "Valve 9"=FALSE, "Valve 10"=FALSE, "Valve 11"=FALSE, "Valve 12"=FALSE, "Valve 13"=FALSE, "Valve 14"=FALSE, "Valve 15"=FALSE, "Valve 16"=FALSE, "Valve 17"=FALSE, "Valve 18"=FALSE, "Valve 19"=FALSE, "Valve 20"=FALSE, "Valve 21"=FALSE, "Valve 22"=FALSE, "Valve 23"=FALSE, "Valve 24"=FALSE, "Valve 25"=FALSE, "Valve 26"=FALSE, "Valve 27"=FALSE, "Valve 28"=FALSE, "Valve 29"=FALSE, "Valve 30"=FALSE, "Valve 31"=FALSE, "Valve 32"=FALSE, "Valve 33"=FALSE, "Valve 34"=FALSE, "Valve 35"=FALSE, "Valve 36"=FALSE, "Valve 37"=FALSE, "Valve 38"=FALSE, "Valve 39"=FALSE, "Valve 40"=FALSE, "Valve 41"=FALSE, "Valve 42"=FALSE, "Valve 43"=FALSE, "Valve 44"=FALSE, "Valve 45"=FALSE, "Valve 46"=FALSE, "Valve 47"=FALSE, "Valve 48"=FALSE, "Valve 49"=FALSE, "Valve 50"=FALSE, "Valve 51"=FALSE, "Valve 52"=FALSE, "Valve 53"=FALSE, "Valve 54"=FALSE, "Valve 55"=FALSE, "Valve 56"=FALSE} ("Water Valves Cluster"), "Valve 56"=TRUE ("Valve 1")) -> (w1511:T8)
                  }
                  frame "Drying Clothes 2" {
                    n451 = Bundle By Name(cluster=T8 {"Valve 1"=FALSE, "Valve 2"=FALSE, "Valve 3"=FALSE, "Valve 4"=FALSE, "Valve 5"=FALSE, "Valve 6"=FALSE, "Valve 7"=FALSE, "Valve 8"=FALSE, "Valve 9"=FALSE, "Valve 10"=FALSE, "Valve 11"=FALSE, "Valve 12"=FALSE, "Valve 13"=FALSE, "Valve 14"=FALSE, "Valve 15"=FALSE, "Valve 16"=FALSE, "Valve 17"=FALSE, "Valve 18"=FALSE, "Valve 19"=FALSE, "Valve 20"=FALSE, "Valve 21"=FALSE, "Valve 22"=FALSE, "Valve 23"=FALSE, "Valve 24"=FALSE, "Valve 25"=FALSE, "Valve 26"=FALSE, "Valve 27"=FALSE, "Valve 28"=FALSE, "Valve 29"=FALSE, "Valve 30"=FALSE, "Valve 31"=FALSE, "Valve 32"=FALSE, "Valve 33"=FALSE, "Valve 34"=FALSE, "Valve 35"=FALSE, "Valve 36"=FALSE, "Valve 37"=FALSE, "Valve 38"=FALSE, "Valve 39"=FALSE, "Valve 40"=FALSE, "Valve 41"=FALSE, "Valve 42"=FALSE, "Valve 43"=FALSE, "Valve 44"=FALSE, "Valve 45"=FALSE, "Valve 46"=FALSE, "Valve 47"=FALSE, "Valve 48"=FALSE, "Valve 49"=FALSE, "Valve 50"=FALSE, "Valve 51"=FALSE, "Valve 52"=FALSE, "Valve 53"=FALSE, "Valve 54"=FALSE, "Valve 55"=FALSE, "Valve 56"=FALSE} ("Water Valves Cluster"), "Valve 56"=TRUE ("Valve 1")) -> (w1515:T8)
                  }
                  frame "Sending Start Stop CMD" {
                    n452 = Bundle By Name(cluster=T9 {"Start Button 21"=FALSE, "Start Button 22"=FALSE, "Start Button 23"=FALSE, "Start Button 24"=FALSE, "Start Button 25"=FALSE, "Start Button 26"=FALSE, "Start Button 27"=FALSE, "Start Button 28"=FALSE, "Start Button 29"=FALSE, "Start Button 30"=FALSE, "Start Button 31"=FALSE, "Start Button 32"=FALSE, "Start Button 33"=FALSE, "Start Button 34"=FALSE, "Start Button 35"=FALSE, "Start Button 36"=FALSE, "Start Button 37"=FALSE, "Start Button 38"=FALSE, "Start Button 39"=FALSE, "Start Button 40"=FALSE, "Start Button 41"=FALSE, "Start Button 42"=FALSE, "Start Button 43"=FALSE, "Start Button 44"=FALSE, "Start Button 12"=FALSE, "Start Button 11"=FALSE, "Start Button 10"=FALSE, "Start Button 9"=FALSE, "Start Button 8"=FALSE, "Start Button 7"=FALSE, "Start Button 6"=FALSE, "Start Button 5"=FALSE, "Start Button 4"=FALSE, "Start Button 3"=FALSE, "Start Button 2"=FALSE, "Start Button 1"=FALSE, "Start Button 20"=FALSE, "Start Button 19"=FALSE, "Start Button 18"=FALSE, "Start Button 17"=FALSE, "Start Button 16"=FALSE, "Start Button 15"=FALSE, "Start Button 14"=FALSE, "Start Button 13"=FALSE, "Start Button 45"=FALSE, "Start Button 46"=FALSE, "Start Button 47"=FALSE, "Start Button 48"=FALSE, "Start Button 49"=FALSE, "Start Button 50"=FALSE, "Start Button 51"=FALSE, "Start Button 52"=FALSE, "Start Button 53"=FALSE, "Start Button 54"=FALSE, "Start Button 55"=FALSE, "Start Button 56"=FALSE} ("Start Buttons Cluster"), "Start Button 56"=TRUE ("Start Button 21")) -> (w1519:T9)
                  }
                  frame "Sending Start Stop CMD 2" {
                    n453 = Bundle By Name(cluster=T9 {"Start Button 21"=FALSE, "Start Button 22"=FALSE, "Start Button 23"=FALSE, "Start Button 24"=FALSE, "Start Button 25"=FALSE, "Start Button 26"=FALSE, "Start Button 27"=FALSE, "Start Button 28"=FALSE, "Start Button 29"=FALSE, "Start Button 30"=FALSE, "Start Button 31"=FALSE, "Start Button 32"=FALSE, "Start Button 33"=FALSE, "Start Button 34"=FALSE, "Start Button 35"=FALSE, "Start Button 36"=FALSE, "Start Button 37"=FALSE, "Start Button 38"=FALSE, "Start Button 39"=FALSE, "Start Button 40"=FALSE, "Start Button 41"=FALSE, "Start Button 42"=FALSE, "Start Button 43"=FALSE, "Start Button 44"=FALSE, "Start Button 12"=FALSE, "Start Button 11"=FALSE, "Start Button 10"=FALSE, "Start Button 9"=FALSE, "Start Button 8"=FALSE, "Start Button 7"=FALSE, "Start Button 6"=FALSE, "Start Button 5"=FALSE, "Start Button 4"=FALSE, "Start Button 3"=FALSE, "Start Button 2"=FALSE, "Start Button 1"=FALSE, "Start Button 20"=FALSE, "Start Button 19"=FALSE, "Start Button 18"=FALSE, "Start Button 17"=FALSE, "Start Button 16"=FALSE, "Start Button 15"=FALSE, "Start Button 14"=FALSE, "Start Button 13"=FALSE, "Start Button 45"=FALSE, "Start Button 46"=FALSE, "Start Button 47"=FALSE, "Start Button 48"=FALSE, "Start Button 49"=FALSE, "Start Button 50"=FALSE, "Start Button 51"=FALSE, "Start Button 52"=FALSE, "Start Button 53"=FALSE, "Start Button 54"=FALSE, "Start Button 55"=FALSE, "Start Button 56"=FALSE} ("Start Buttons Cluster"), "Start Button 56"=TRUE ("Start Button 21")) -> (w1522:T9)
                  }
                  frame "Sending Start Stop CMD 3" {
                    n454 = Bundle By Name(cluster=T9 {"Start Button 21"=FALSE, "Start Button 22"=FALSE, "Start Button 23"=FALSE, "Start Button 24"=FALSE, "Start Button 25"=FALSE, "Start Button 26"=FALSE, "Start Button 27"=FALSE, "Start Button 28"=FALSE, "Start Button 29"=FALSE, "Start Button 30"=FALSE, "Start Button 31"=FALSE, "Start Button 32"=FALSE, "Start Button 33"=FALSE, "Start Button 34"=FALSE, "Start Button 35"=FALSE, "Start Button 36"=FALSE, "Start Button 37"=FALSE, "Start Button 38"=FALSE, "Start Button 39"=FALSE, "Start Button 40"=FALSE, "Start Button 41"=FALSE, "Start Button 42"=FALSE, "Start Button 43"=FALSE, "Start Button 44"=FALSE, "Start Button 12"=FALSE, "Start Button 11"=FALSE, "Start Button 10"=FALSE, "Start Button 9"=FALSE, "Start Button 8"=FALSE, "Start Button 7"=FALSE, "Start Button 6"=FALSE, "Start Button 5"=FALSE, "Start Button 4"=FALSE, "Start Button 3"=FALSE, "Start Button 2"=FALSE, "Start Button 1"=FALSE, "Start Button 20"=FALSE, "Start Button 19"=FALSE, "Start Button 18"=FALSE, "Start Button 17"=FALSE, "Start Button 16"=FALSE, "Start Button 15"=FALSE, "Start Button 14"=FALSE, "Start Button 13"=FALSE, "Start Button 45"=FALSE, "Start Button 46"=FALSE, "Start Button 47"=FALSE, "Start Button 48"=FALSE, "Start Button 49"=FALSE, "Start Button 50"=FALSE, "Start Button 51"=FALSE, "Start Button 52"=FALSE, "Start Button 53"=FALSE, "Start Button 54"=FALSE, "Start Button 55"=FALSE, "Start Button 56"=FALSE} ("Start Buttons Cluster"), "Start Button 56"=TRUE ("Start Button 21")) -> (w1526:T9)
                  }
                }
              }
            }
            n455 = local write "Water Valves Cluster"(w178) -> ()
            n456 = local write "Start Buttons Cluster"(w177) -> ()
            n457 = Bundle By Name(cluster=w182, "Water Valves Cluster"=w178, "Start Buttons Cluster"=w177) -> (w181:T14)
          }
          frame "Operate As Stand-Alone EXE" {
            w1531 = T9 {"Start Button 21"=FALSE, "Start Button 22"=FALSE, "Start Button 23"=FALSE, "Start Button 24"=FALSE, "Start Button 25"=FALSE, "Start Button 26"=FALSE, "Start Button 27"=FALSE, "Start Button 28"=FALSE, "Start Button 29"=FALSE, "Start Button 30"=FALSE, "Start Button 31"=FALSE, "Start Button 32"=FALSE, "Start Button 33"=FALSE, "Start Button 34"=FALSE, "Start Button 35"=FALSE, "Start Button 36"=FALSE, "Start Button 37"=FALSE, "Start Button 38"=FALSE, "Start Button 39"=FALSE, "Start Button 40"=FALSE, "Start Button 41"=FALSE, "Start Button 42"=FALSE, "Start Button 43"=FALSE, "Start Button 44"=FALSE, "Start Button 12"=FALSE, "Start Button 11"=FALSE, "Start Button 10"=FALSE, "Start Button 9"=FALSE, "Start Button 8"=FALSE, "Start Button 7"=FALSE, "Start Button 6"=FALSE, "Start Button 5"=FALSE, "Start Button 4"=FALSE, "Start Button 3"=FALSE, "Start Button 2"=FALSE, "Start Button 1"=FALSE, "Start Button 20"=FALSE, "Start Button 19"=FALSE, "Start Button 18"=FALSE, "Start Button 17"=FALSE, "Start Button 16"=FALSE, "Start Button 15"=FALSE, "Start Button 14"=FALSE, "Start Button 13"=FALSE, "Start Button 45"=FALSE, "Start Button 46"=FALSE, "Start Button 47"=FALSE, "Start Button 48"=FALSE, "Start Button 49"=FALSE, "Start Button 50"=FALSE, "Start Button 51"=FALSE, "Start Button 52"=FALSE, "Start Button 53"=FALSE, "Start Button 54"=FALSE, "Start Button 55"=FALSE, "Start Button 56"=FALSE} ("Start Buttons Cluster")
            w1530 = T8 {"Valve 1"=FALSE, "Valve 2"=FALSE, "Valve 3"=FALSE, "Valve 4"=FALSE, "Valve 5"=FALSE, "Valve 6"=FALSE, "Valve 7"=FALSE, "Valve 8"=FALSE, "Valve 9"=FALSE, "Valve 10"=FALSE, "Valve 11"=FALSE, "Valve 12"=FALSE, "Valve 13"=FALSE, "Valve 14"=FALSE, "Valve 15"=FALSE, "Valve 16"=FALSE, "Valve 17"=FALSE, "Valve 18"=FALSE, "Valve 19"=FALSE, "Valve 20"=FALSE, "Valve 21"=FALSE, "Valve 22"=FALSE, "Valve 23"=FALSE, "Valve 24"=FALSE, "Valve 25"=FALSE, "Valve 26"=FALSE, "Valve 27"=FALSE, "Valve 28"=FALSE, "Valve 29"=FALSE, "Valve 30"=FALSE, "Valve 31"=FALSE, "Valve 32"=FALSE, "Valve 33"=FALSE, "Valve 34"=FALSE, "Valve 35"=FALSE, "Valve 36"=FALSE, "Valve 37"=FALSE, "Valve 38"=FALSE, "Valve 39"=FALSE, "Valve 40"=FALSE, "Valve 41"=FALSE, "Valve 42"=FALSE, "Valve 43"=FALSE, "Valve 44"=FALSE, "Valve 45"=FALSE, "Valve 46"=FALSE, "Valve 47"=FALSE, "Valve 48"=FALSE, "Valve 49"=FALSE, "Valve 50"=FALSE, "Valve 51"=FALSE, "Valve 52"=FALSE, "Valve 53"=FALSE, "Valve 54"=FALSE, "Valve 55"=FALSE, "Valve 56"=FALSE} ("Water Valves Cluster")
            n458 = local write "Start Buttons Cluster"(w1531) -> ()
            n459 = local write "Water Valves Cluster"(w1530) -> ()
            n460 = Bundle By Name(cluster=w1533, "Start Buttons Cluster"=w1531, "Water Valves Cluster"=w1530) -> (w1532:T14)
          }
        }
        n461 = for {
          tunnel: w173 -> [w1539] mode=indexing
          tunnel: [w1538] -> w170 mode=indexing
          tunnel: [w1534] -> w171 mode=indexing
          n462 = Unbundle By Name(w1539) -> ("Agilent Station"=w1537:string, "Channel"=w1538:string)
          n463 = Decimal String To Number(string=w1537) -> (number=w1536:i32)  [unwired: 2 in, 1 out]
          n464 = To Unsigned Byte Integer(number=w1536) -> (unsigned 8bit integer=w1535:u8)
          n465 = call "WILT Agilent Ref Type Conversion.vi"("Agilent Ref"=w1535) -> ("VISA resource name"=w1534:refnum<visa-resource-name>)  [unwired: 14 in]
        }
        "Agilent Array" <- w171
        "Agilent Channels" <- w170
        n466 = Bundle By Name(cluster=w167, "Agilent Array"=w171, "Agilent Channel Array"=w170) -> (w172:T14)
        n467 = call <vilib>:"Add State(s) to Queue__jki_lib_state_machine.vi"("State(s) in (\"\")"=w176) -> ("States Out"=w175:string)  [unwired: 14 in]
      }
      frame "UI: Cursor Set" {
        # "Argument"
        # "Set and Unset Cursor Busy.\n(Usage: \"UI: Cursor Set >> Busy|Idle\")"
        n468 = case shown="\"Idle\", Default" w1540 {
          tunnel: w1542 -> [w1547 w1549]
          tunnel: [w1546 w1548] -> w1541
          frame "Idle", Default {
            n469 = call <vilib>:"Unset Busy.vi"("error in (no error)"=w1547) -> ("error out"=w1546:errorcluster)  [unwired: 10 in]
          }
          frame "Busy" {
            n470 = call <vilib>:"Set Busy.vi"("error in (no error)"=w1549) -> ("error out"=w1548:errorcluster)  [unwired: 9 in, 1 out]
          }
        }
        n471 = call <vilib>:"Add State(s) to Queue__jki_lib_state_machine.vi"("State(s) in (\"\")"=w1545) -> ("States Out"=w1544:string)  [unwired: 14 in]
      }
      frame "UI: Front Panel State" {
        # "Argument"
        # "Set Front Panel Open or Closed\n(Usage: \"UI: Front Panel State >> Open|Close\")"
        n472 = Unbundle By Name(w1552) -> ("Core.Current VI Reference"=w1551:refnum<vi>)
        n473 = case shown="\"Open\", Default" w1550 {
          tunnel: w1554 -> [w1560 w1573]
          tunnel: [w1562 w1574] -> w1553
          tunnel: w1551 -> [w1561 w1571]
          frame "Open", Default {
            n474 = property class="VI"(reference=w1561, error in=w1560) -> (reference out=w1558:refnum<vi>, error out=w1559:errorcluster, "Front Panel.Open"=w1557:bool)
            n475 = case shown="False" w1557 {
              tunnel: [w1565 w1568] -> w1562
              tunnel: w1559 -> [w1564 w1568]
              tunnel: w1558 -> [w1563 _]
              frame False {
                n476 = invoke class="VI" method="FP.Open"(reference=w1563, error in=w1564, "Activate"=TRUE, "State"=T13."Standard") -> (error out=w1565:errorcluster)  [unwired: 1 in, 4 out]
              }
              frame True {
              }
            }
          }
          frame "Close" {
            n477 = property class="VI"(reference=w1571, error in=w1573) -> (reference out=w1570:refnum<vi>, error out=w1572:errorcluster, "Front Panel.Open"=w1569:bool)
            n478 = case shown="True" w1569 {
              tunnel: [w1575 w1578] -> w1574
              tunnel: w1572 -> [w1575 w1577]
              tunnel: w1570 -> [_ w1576]
              frame False {
              }
              frame True {
                n479 = invoke class="VI" method="FP.Close"(reference=w1576, error in=w1577) -> (error out=w1578:errorcluster)  [unwired: 1 in, 2 out]
              }
            }
          }
        }
        n480 = call <vilib>:"Add State(s) to Queue__jki_lib_state_machine.vi"("State(s) in (\"\")"=w1556) -> ("States Out"=w1555:string)  [unwired: 14 in]
      }
      frame "---------- Macro ----------" {
        # "Do not put any code in this frame.\n(It is a separator no-op. You can make a copy of this frame to create a new Macro frame)"
        n481 = call <vilib>:"Add State(s) to Queue__jki_lib_state_machine.vi"("State(s) in (\"\")"=w1582) -> ("States Out"=w1581:string)  [unwired: 14 in]
      }
      frame "Macro: Initialize" {
        w1583 = "Data: Initialize\nAgilent Channels\nInitialize Core Data\nUI: Initialize\nUI: Front Panel State >> Open\nBuild Button Array"  # Data: Initialize Agilent Channels Initialize Core Data UI: Initialize UI: Front Panel State >> Open Build Button Array
        # "Shuts all valves in beginning, so they are in known state."
        # "Initialization Macro\n(This is called once, when the VI starts)"
        n482 = call <vilib>:"Add State(s) to Queue__jki_lib_state_machine.vi"("State(s) in Front (\"\")"=w1583, "State(s) in (\"\")"=w1587) -> ("States Out"=w1586:string)  [unwired: 13 in]
      }
      frame "Macro: Exit" {
        # "Exit Macro\n(This is called once, when the VI exits)"
        n483 = Unbundle By Name(w1594) -> ("Core.Close Panel on Exit?"=w1593:bool)
        n484 = Select(t="UI: Front Panel State >> Close", s=w1593, f="") -> (s? t:f=w1590:string)
        n485 = call <vilib>:"Add State(s) to Queue__jki_lib_state_machine.vi"("State(s) in (\"\")"=w1590, "State(s) at Back (\"\")"="Data: Cleanup\nExit") -> ("States Out"=w1588:string)  [unwired: 13 in]
        n486 = call <vilib>:"Add State(s) to Queue__jki_lib_state_machine.vi"("State(s) in Front (\"\")"=w1588, "State(s) in (\"\")"=w1597) -> ("States Out"=w1596:string)  [unwired: 13 in]
      }
      frame "---------- New Category ----------" {
        # "Template Separator\n(You can make a copy of, or modify, this frame)"
        n487 = call <vilib>:"Add State(s) to Queue__jki_lib_state_machine.vi"("State(s) in (\"\")"=w1601) -> ("States Out"=w1600:string)  [unwired: 14 in]
      }
      frame "Select Valve" {
        n488 = Unbundle By Name(w1612) -> ("Agilent Switches"=w1607:T2[], "Station Test State In"=w1608:T5)
        n489 = disable-structure shown="Enabled" {
          disable-tunnel: w1608 -> [w1619 _]
          frame Enabled {
            n490 = local read "Operation Type"() -> (w1618:T11)
            n491 = case shown="\"Operate As SubVI\", Default" w1618 {
              tunnel: w1619 -> [w1622 _]
              frame "Operate As SubVI", Default {
                n492 = local read "Station Number"() -> (w1621:i32)
                n493 = call "WILT Number of Button Presses.vi"("Station Number"=w1621, "Station Test State In"=w1622) -> ("Number of ON/OFF Cycles"=w1620:i32)  [unwired: 9 in]
                n494 = local write "Number of ON/OFF Cycles"(w1620) -> ()
              }
              frame "Operate As Stand-Alone EXE" {
              }
            }
          }
          frame Disabled {
          }
        }
        n495 = local read "Start Buttons Cluster"() -> (w1604:T9)
        n496 = local read "Water Valves Cluster"() -> (w1605:T8)
        n497 = call "WILT Search For Valve Channel.vi"("Start Buttons Cluster"=w1604, "Water Valves Cluster"=w1605, "Agilent Valve and Switch Locations"=w1607) -> ("Channel"=w1602:string, "Agilent Station"=w1603:string, "Label"=→"Label":string)  [unwired: 5 in, 1 out]
        "Agilent Used" <- w1603
        "Channel Being Used" <- w1602
        n498 = Decimal String To Number(string=w1603) -> (number=w1613:i32)  [unwired: 2 in, 1 out]
        n499 = To Unsigned Byte Integer(number=w1613) -> (unsigned 8bit integer=w1614:u8)
